vi "Data Lookup Table Set Signals (Range).vi"(8 "error in (no error)":errorcluster, 9 "Signals":dbl[](array[numeric]), 10 "Direct Access":cluster{"Offset":u32, "Length":u32}, 11 "Data Ref":refnum<data-value>) -> (0 "error out":errorcluster {"code" min=0 max=0}, 3 "Data Ref out":refnum<data-value>)   [LabVIEW 2013, in "J1939 Addon Engine.lvlib"]
uses:
  J1939 Addon Engine.lvlib
  Diagnostics Addon/Source/Engine/SubVIs/Datatable Lookup DVR.ctl
  Types/Data Lookup Table Action.ctl
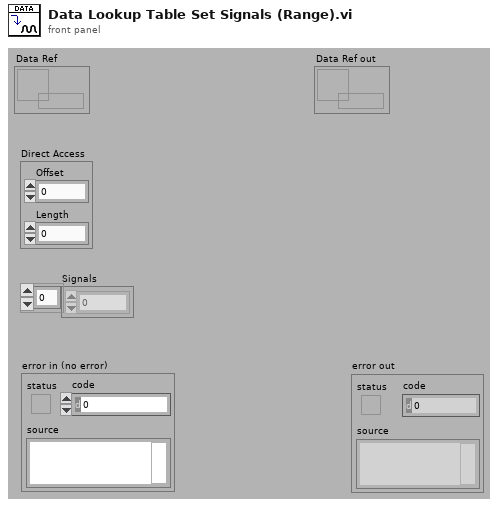
[diagram p1: front panel]
types:
  T1 = typedef "J1939 Addon Engine.lvlib/Data Lookup Table Action.ctl" = enum16{"Get All", "Set All", "Set Frame", "Get Frame", "Set Range", "Get Range"}
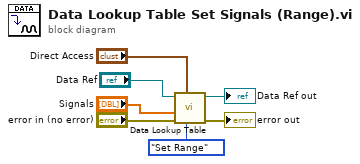
[diagram p0: block diagram]
diagram:
  n1 = call "Data Lookup Table.vi"("command"=Data_Lookup_Table_Action."Set Range", "Direct Access"="Direct Access", "error in (no error)"="error in (no error)", "Signals"="Signals", "DVR Ref"="Data Ref") -> ("error out"=→"error out":errorcluster, "DVR Ref out"=→"Data Ref out":refnum<data-value>)  [unwired: 4 in, 1 out]
